vi "modbus-parameter-to-float.vi"(1 "MODBUS parameter":u16[](array[numeric]) format="%x") -> (0 "float":sgl[](array[numeric]))   [LabVIEW 2016]
doc: "Input: array (length=2) given by Modbus\nThis VI converts\n1 Parameter = 2 Words = 4 Bytes --> 32-bit real\nKeep in mind, that the hexadecimal bytes given by Modbus have to be reversed for conversion!!!"
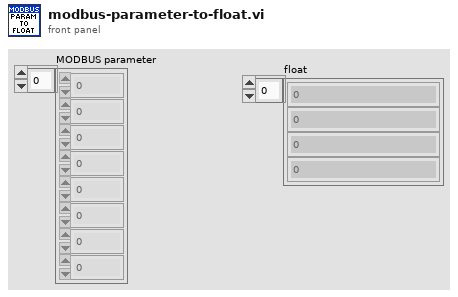
[diagram p1: front panel]
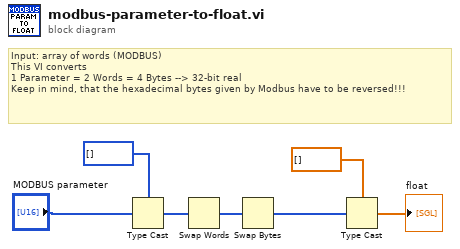
[diagram p0: block diagram]
diagram:
  # "Input: array of words (MODBUS)\nThis VI converts\n1 Parameter = 2 Words = 4 Bytes --> 32-bit real\nKeep in mind, that the hexadecimal bytes given by Modbus have to be reversed!!!"
  n1 = Type Cast(type=i32[] [], x="MODBUS parameter") -> (*(type *) &x=w6:i32[])
  n2 = Swap Words(1:w6) -> (0:w3:i32[])
  n3 = Swap Bytes(anything=w3) -> (byte swapped=w2:i32[])
  n4 = Type Cast(type=sgl[] [], x=w2) -> (*(type *) &x=→"float":sgl[])
